vi "BinDP-Zoom Spectrum.vi"(7 "DP window":refnum<vi>, 8 "error in (no error)":errorcluster, 9 "Width (kHz)":dbl=4.0, 11 "DP Freqs":T1) -> (0 "error out":errorcluster)   [LabVIEW 2020]
uses:
  Typedefs/DP-Freqs.ctl
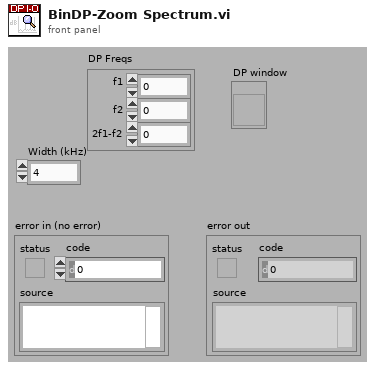
[diagram p1: front panel]
types:
  T1 = typedef "DP-Freqs.ctl" = cluster{"f1":dbl, "f2":dbl, "2f1-f2":dbl}
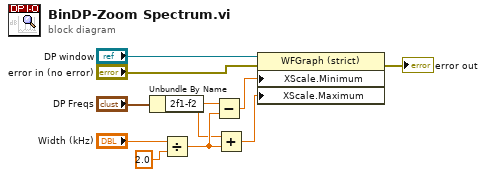
[diagram p0: block diagram]
diagram:
  n1 = Unbundle By Name("DP Freqs") -> ("2f1-f2"=w2:dbl)
  n2 = Divide(x="Width (kHz)", y=2.0) -> (x/y=w6:dbl)
  n3 = Subtract(x=w2, y=w6) -> (x-y=w5:dbl)
  n4 = Add(x=w2, y=w6) -> (x+y=w4:dbl)
  n5 = property class="WFGraph (strict)"(reference="DP window", error in="error in (no error)", "XScale.Minimum"=w5, "XScale.Maximum"=w4) -> (error out=→"error out":errorcluster)  [unwired: 1 out]
